vi "ExtractName.vi"(0 "Full File Name":string) -> (1 "Root File Name":string, 2 "File Number":string, 3 "Digits in File Number":i32)   [LabVIEW 2022 SP3]
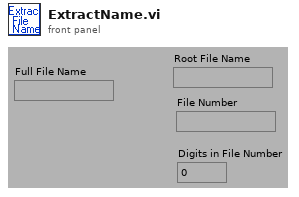
[diagram p1: front panel]
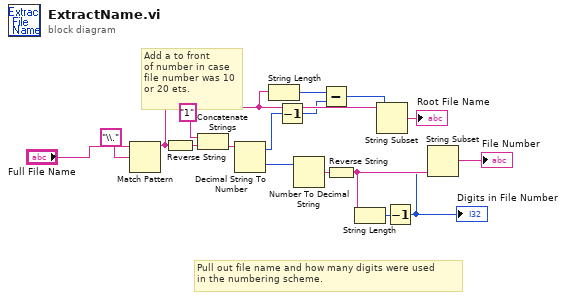
[diagram p0: block diagram]
diagram:
  # "Add a to front\nof number in case\nfile number was 10\nor 20 ets."
  # "Pull out file name and how many digits were used \nin the numbering scheme."
  n1 = Match Pattern(string="Full File Name", regular expression="\\." ("string")) -> (before substring=w11:string)  [unwired: 4 out]
  n2 = Reverse String(1:w11) -> (0:w5:string)
  n3 = Concatenate Strings("1", w5) -> (w7:string)
  n4 = Decimal String To Number(string=w7) -> (offset past number=w13:i32, number=w15:i32)  [unwired: 2 out]
  n5 = String Length(string=w11) -> (length=w14:i32)
  n6 = Decrement(x=w13) -> (x-1=w1:i32)
  n7 = Number To Decimal String(number=w15) -> (decimal integer string=w16:string)  [unwired: 1 out]
  n8 = Subtract(x=w14, y=w1) -> (x-y=w12:i32)
  n9 = Reverse String(1:w16) -> (0:w4:string)
  n10 = String Length(string=w4) -> (length=w8:i32)
  n11 = String Subset(string=w11, length (rest)=w12) -> (substring=→"Root File Name":string)  [unwired: 1 out]
  n12 = Decrement(x=w8) -> (x-1=w2:i32)
  "Digits in File Number" <- w2
  n13 = String Subset(string=w4, length (rest)=w2) -> (substring=→"File Number":string)  [unwired: 1 out]
